vi "Dequeue DI Data.vi"(11 "error in (no error)":errorcluster) -> (10 "DI Waveforms":bool[][](array[boolean]), 15 "error out":errorcluster)   [LabVIEW 2020]
uses:
  DAQ Engine VIs/PXI Globals.vi
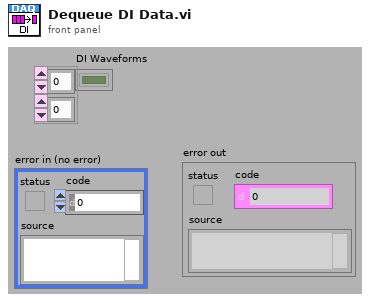
[diagram p1: front panel]
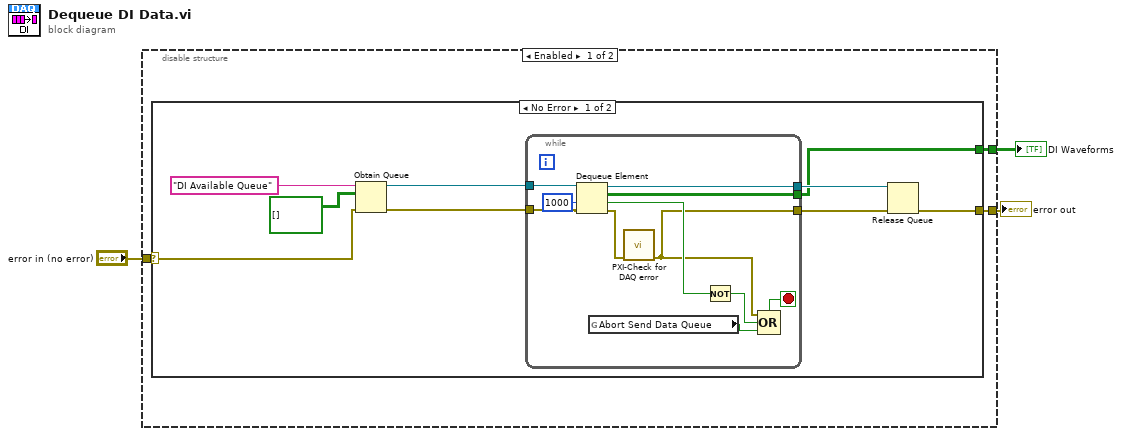
[diagram p0: block diagram]
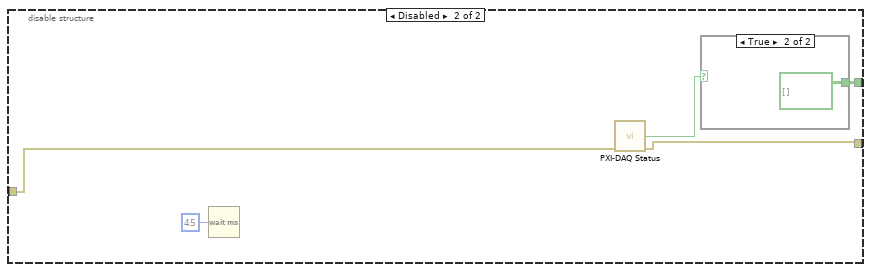
[diagram p3: hidden frame]
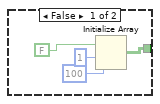
[diagram p4: hidden frame]
diagram:
  n1 = disable-structure shown="Enabled" {
    disable-tunnel: [w6 w29] -> w3
    disable-tunnel: "error in (no error)" -> [w5 w30]
    disable-tunnel: [w4 w31] -> w1
    frame Enabled {
      n2 = case shown="No Error" w5 {
        selector: w5 -> [w9 w27]
        tunnel: [w14 w27] -> w6
        tunnel: [w7 _] -> w4
        frame No Error {
          n3 = Obtain Queue(name (unnamed)="DI Available Queue", element data type=bool[][] [] ("AI Waveforms 2"), error in (no error)=w9) -> (queue out=w11:refnum<queue>, error out=w8:errorcluster)  [unwired: 2 in, 1 out]
          n4 = while {
            tunnel: [w16] -> w15
            tunnel: w11 -> [w26]
            tunnel: [w25] -> w7
            tunnel: [w24] -> w10
            tunnel: w8 -> [w17]
            stop <- w19 stop-if-true
            n5 = Dequeue Element(queue=w26, timeout in ms (-1)=1000, error in (no error)=w17) -> (queue out=w24:refnum<queue>, element=w25:bool[][], timed out?=w21:bool, error out=w18:errorcluster)
            n6 = global read "PXI Globals.vi" "Abort Send Data Queue"() -> (w22:bool)
            n7 = call "PXI-Check for DAQ error.vi"("error in (no error)"=w18) -> ("error out"=w16:errorcluster)  [unwired: 14 in]
            n8 = Not(x=w21) -> (.not. x?=w20:bool)
            n9 = Compound Arithmetic op=OR(w16, w20, w22) -> (w19:bool)
          }
          n10 = Release Queue(queue=w10, error in (no error)=w15) -> (error out=w14:errorcluster)  [unwired: 1 in, 2 out]
        }
        frame Error {
        }
      }
    }
    frame Disabled {
      n11 = Wait (ms)(milliseconds to wait=u32 45) -> ()  [unwired: 1 out]
      n12 = call "PXI-DAQ Status.vi"("error in (no error)"=w30) -> ("Finished?"=w28:bool, "error out"=w29:errorcluster)  [unwired: 13 in]
      n13 = case shown="True" w28 {
        tunnel: [w35 bool[][] []] -> w31
        frame False {
          n14 = Initialize Array(FALSE, 1 ("dimension size"), 100 ("dimension size")) -> (w35:bool[][])
        }
        frame True {
        }
      }
    }
  }
  "error out" <- w3
  "DI Waveforms" <- w1
